vi "2-D TimeStamped Logging (SubVI) v0.1.vi"(8 "error in (no error)":errorcluster, 10 "array":dbl[](array[numeric]), 11 "path":path) -> (0 "error out":errorcluster)   [LabVIEW 2018]
uses:
  <vilib>/Utility/file.llb/Write Delimited Spreadsheet (string).vi
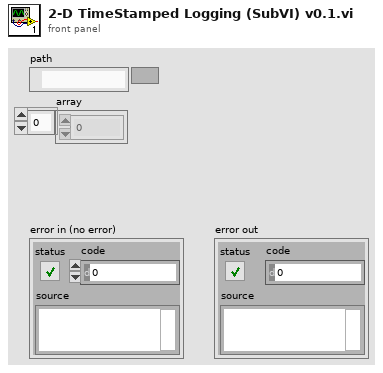
[diagram p1: front panel]
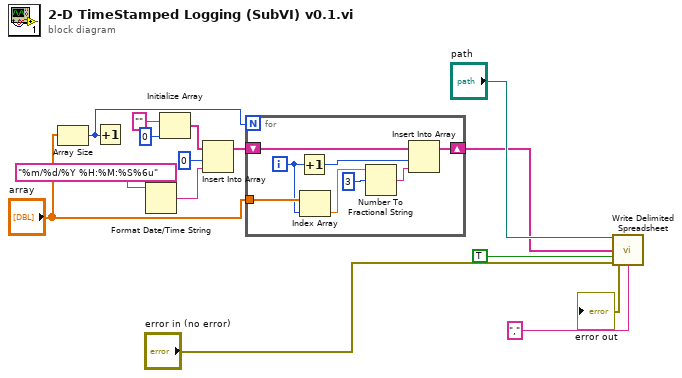
[diagram p0: block diagram]
diagram:
  n1 = Array Size(array="array") -> (size(s)=w8:i32)
  n2 = Increment(x=w8) -> ()  [unwired: 1 out]
  n3 = Format Date/Time String(time format string (%c)="%m/%d/%Y %H:%M:%S%6u") -> (date/time string=w5:string)  [unwired: 2 in]
  n4 = Initialize Array("" ("element"), 0 ("dimension size")) -> (w7:string[])
  n5 = Insert Into Array(array=w7, index=0, new element=w5) -> (w3:string[])
  n6 = for {
    N: w8 -> [_]
    tunnel: "array" -> [w23]
    shift-right: [w18] -> w4
    shift-left: w3 -> [w19]
    i -> [w16]
    n7 = Increment(x=w16) -> (x+1=w17:i32)
    n8 = Index Array(array=w23, index=w16) -> (element=w21:dbl)
    n9 = Number To Fractional String(number=w21, width (-)=i16 3) -> (F-format string=w20:string)  [unwired: 2 in]
    n10 = Insert Into Array(array=w19, index=w17, new element=w20) -> (w18:string[])
  }
  n11 = call-poly <vilib>:"Write Delimited Spreadsheet.vi"("file path (dialog if empty)"="path", "1D data"=w4, "append to file? (new file:F)"=TRUE, "error in (no error)"="error in (no error)", "delimiter (\\t)"="," ("delimiter (\\t)")) -> ("error out"=→"error out":errorcluster)  [unwired: 9 in, 1 out]
